vi "Do.vi"(8 "error in (no error)":errorcluster, 9 "Events":refnum<class "Events.lvclass">, 10 "Message Loop Data in":T1, 11 "IPublish in":refnum<class "IPublish.lvclass">) -> (0 "error out":errorcluster, 1 "Write request":T10, 2 "Message Loop Data out":T1, 3 "IPublish out":refnum<class "IPublish.lvclass">)   [LabVIEW 2020, in "wamplv.lvlib" / "IPublish.lvclass"]
uses:
  IPublish.lvclass
  WAMP Client/API/TypeDefs/WAMP error (JSON).ctl
  wamplv.lvlib
  WAMP Client/API/TypeDefs/Combined error.ctl
  WAMP Client/Private/TypeDef/Success or error (JSON).ctl
  WAMP Client/Private/TypeDef/Publish Requests Map.ctl
  WAMP Client/Private/TypeDef/Endpoint Data.ctl
  Call/ICallRequest/ICallRequest.lvclass
  WAMP Client/Private/TypeDef/CALL Request Map.ctl
  WAMP Client/Private/TypeDef/SUBSCRIBE Requests Map.ctl
  WAMP Client/Private/TypeDef/Subscriptions Map.ctl
  WAMP Client/Private/TypeDef/Unsubscribe Requests Map.ctl
  WAMP Client/Private/TypeDef/Unregister request (JSON).ctl
  WAMP Client/Private/TypeDef/Unregister requests map.ctl
  WAMP Client/Private/TypeDef/Message Loop Data.ctl
  TypeDefs/Transport type.ctl
  WAMP Client/Private/TypeDef/Write queue item.ctl
  Events/EventsParent/Events.lvclass
  Subscribe/ISubscribe/ISubscribe.lvclass
  Message loop classes/Subscription details/SubscriptionDetailsParent/SubscriptionDetailsParent.lvclass
  Unsubscribe/IUnsubscribe/IUnsubscribe.lvclass
  Register/IRegister/IRegister.lvclass
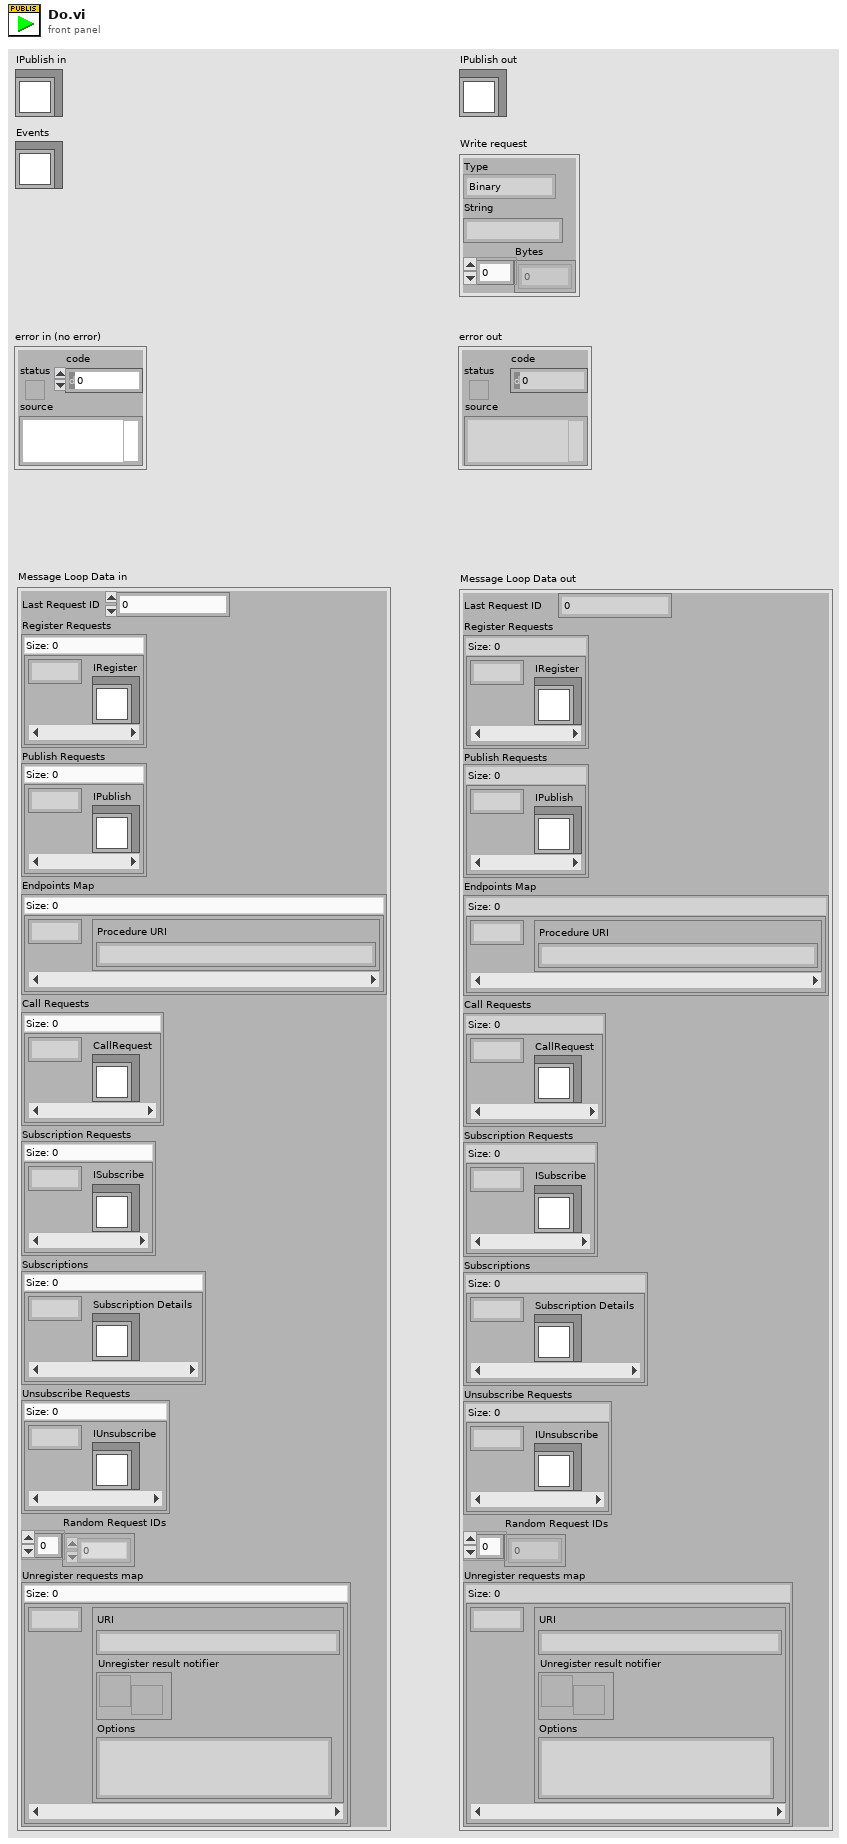
[diagram p1: front panel]
types:
  T1 = typedef "wamplv.lvlib/Message Loop Data.ctl" = cluster{"Last Request ID":u64, "Register Requests":map{u64, refnum<class "IRegister.lvclass">}, "Publish Requests":T2, "Endpoints Map":map{u64, T3}, "Call Requests":T4, "Subscription Requests":T5, "Subscriptions":T6, "Unsubscribe Requests":T7, "Random Request IDs":u64[], "Unregister requests map":T8}
  T2 = typedef "wamplv.lvlib/Publish Requests Map.ctl" = map{u64, refnum<class "IPublish.lvclass">}
  T3 = typedef "wamplv.lvlib/Endpoint Data.ctl" = cluster{"Procedure URI":string}
  T4 = typedef "wamplv.lvlib/CALL Request Map.ctl" = map{u64, refnum<class "ICallRequest.lvclass">}
  T5 = typedef "wamplv.lvlib/SUBSCRIBE Requests Map.ctl" = map{u64, refnum<class "ISubscribe.lvclass">}
  T6 = typedef "wamplv.lvlib/Subscriptions Map.ctl" = map{u64, refnum<class "SubscriptionDetailsParent.lvclass">}
  T7 = typedef "wamplv.lvlib/Unsubscribe Requests Map.ctl" = map{u64, refnum<class "IUnsubscribe.lvclass">}
  T8 = typedef "wamplv.lvlib/Unregister requests map.ctl" = map{u64, T9}
  T9 = typedef "wamplv.lvlib/Unregister request (JSON).ctl" = cluster{"URI":string, "Unregister result notifier":refnum<notifier>, "Options":string}
  T10 = typedef "wamplv.lvlib/Write queue item.ctl" = cluster{"Type":T11, "String":string, "Bytes":u8[]}
  T11 = typedef "wamplv.lvlib/Transport type.ctl" = enum16{"Binary", "Text"}
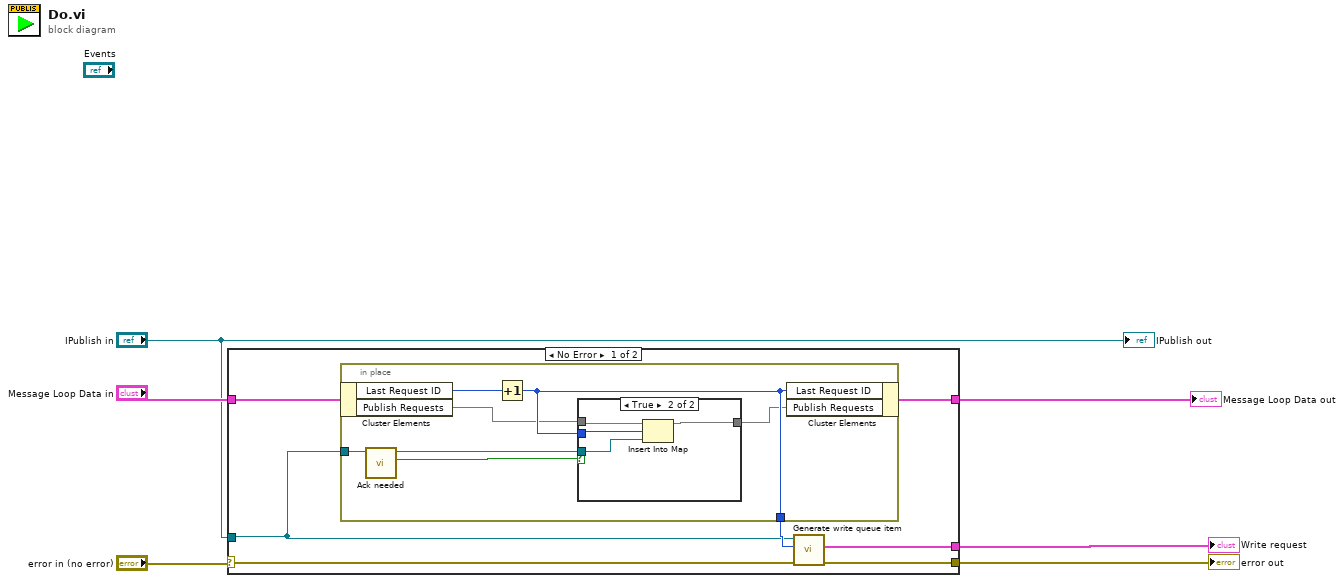
[diagram p0: block diagram]
diagram:
  n1 = case shown="No Error" "error in (no error)" {
    selector: "error in (no error)" -> [w8 w27]
    tunnel: [w11 w27] -> w5
    tunnel: "IPublish in" -> [w7 _]
    tunnel: "Message Loop Data in" -> [w13 w26]
    tunnel: [w12 w26] -> w3
    tunnel: [w10 _] -> w2
    frame No Error {
      n2 = in-place "In Place Element Structure" {
        in-place-border: w7 -> [w16]
        in-place-border: [w19] -> w9
        n3 = in-place-cluster #1(w13) -> ("Last Request ID"=w20:u64, "Publish Requests"=w17:T2)
        n4 = call-dynamic "Ack needed.vi"("IPublish in"=w16) -> ("Ack needed?"=w14:bool, "IPublish out"=w15:refnum<class "IPublish.lvclass">)  [unwired: 9 in]
        n5 = Increment(x=w20) -> (x+1=w19:u64)
        n6 = case shown="True" w14 {
          tunnel: w17 -> [w21 w25]
          tunnel: w15 -> [_ w24]
          tunnel: [w21 w23] -> w18
          tunnel: w19 -> [_ w22]
          frame False {
          }
          frame True {
            n7 = Insert Into Map(map in=w25, key=w22, value=w24) -> (map out=w23:T2)  [unwired: 2 out]
          }
        }
        n8 = in-place-cluster #1("Last Request ID"=w19, "Publish Requests"=w18) -> (w12:T1)
      }
      n9 = call-dynamic "Generate write queue item.vi"("error in (no error)"=w8, "Request ID"=w9, "IPublish in"=w7) -> ("error out"=w11:errorcluster, "Write queue item"=w10:T10)  [unwired: 6 in, 1 out]
    }
    frame Error {
    }
  }
  "error out" <- w5
  "Message Loop Data out" <- w3
  "Write request" <- w2
  "IPublish out" <- "IPublish in"
